vi "unit_length.vi"() -> ()   [LabVIEW 2024]
panel:
  in  "unit length":u32
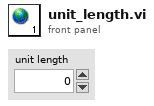
[diagram p1: front panel]
diagram:
